vi "main.vi"(8 "error in (no error)":errorcluster, 9 "enable_event":bool, 10 "max_queue_size":i32=10, 11 "references_queue":refnum<queue>) -> (0 "error out":errorcluster)   [LabVIEW 2015, in "repub-dvr_nre.lvlib"]
doc: "This VI is (a) focal point of the module in the event that there is a need to serialize processes or have loops specific to the module that need to run to aid in the modules major functionality."
uses:
  repub-dvr_nre.lvlib
  public/_controls/references.ctl
  private/_controls/input.ctl
  private/_controls/input_command.ctl
  private/_controls/output.ctl
  private/_controls/data.ctl
  public/_controls/configuration.ctl
  lv-recipe-machine/private/_controls/recipe_data.ctl
  lv-recipe-machine/public/_controls/mode.ctl
  lv-recipe-machine/public/_controls/manual_state.ctl
  lv-recipe-machine/public/_controls/automatic_state.ctl
  <userlib>/antonio-alexander/lv-waitgroup/public/_controls/api_waitgroup.ctl
  lv-recipe-machine/public/_controls/transition.ctl
  public/_controls/change.ctl
  public/_controls/status.ctl
  public/_controls/error.ctl
  lv-recipe-machine/lv-recipe-machine.lvlib
  <userlib>/antonio-alexander/lv-waitgroup/lv-waitgroup.lvlib
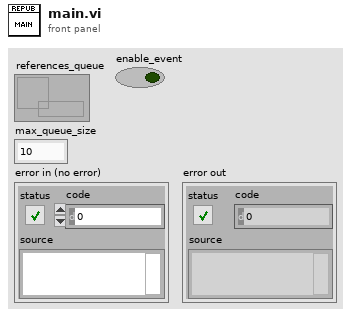
[diagram p1: front panel]
types:
  T1 = typedef "lv-recipe-machine.lvlib/transition.ctl" = cluster{"next_step":string, "data":variant, "error":errorcluster}
  T2 = typedef "repub-dvr_nre.lvlib/references.ctl" = cluster{"semaphore":T3, "input_queue":refnum<queue>, "output_queue":refnum<queue>, "data_dvr":refnum<data-value>, "stop_notifier":refnum<notifier>, "transition_queue":refnum<queue>, "change_in_queue":refnum<queue>, "change_out_queue":refnum<queue>, "status_queue":refnum<queue>, "change_in_event":refnum<user-event>, "change_out_event":refnum<user-event>, "status_event":refnum<user-event>}
  T3 = typedef "Semaphore RefNum" = refnum<k1>
  T4 = typedef "repub-dvr_nre.lvlib/output.ctl" = cluster{"data":variant, "error":errorcluster}
  T5 = typedef "repub-dvr_nre.lvlib/input.ctl" = cluster{"command":T6, "data":variant}
  T6 = typedef "repub-dvr_nre.lvlib/input_command.ctl" = enum8{"<input_command>", "die", "<null>"}
  T7 = typedef "repub-dvr_nre.lvlib/data.ctl" = cluster{"configuration":T8, "working":cluster{"recipe_data":T9, "api_waitgroup":T13}}
  T8 = typedef "repub-dvr_nre.lvlib/configuration.ctl" = cluster{dbl}
  T9 = typedef "lv-recipe-machine.lvlib/recipe_data.ctl" = cluster{"mode":T10, "manual_state":T11, "automatic_state":T12, "step":string, "automatic_recipe":variant, "manual_actions":variant}
  T10 = typedef "lv-recipe-machine.lvlib/mode.ctl" = enum16{"<mode>", "manual", "automatic", "<null>"}
  T11 = typedef "lv-recipe-machine.lvlib/manual_state.ctl" = enum16{"<manual_state>", "failed", "action", "running", "idle", "<null>"}
  T12 = typedef "lv-recipe-machine.lvlib/automatic_state.ctl" = enum16{"<automatic_state>", "failed", "idle", "running", "paused", "transition", "stopped", "<null>"}
  T13 = typedef "lv-waitgroup.lvlib/api_waitgroup.ctl" = cluster{"waitgroups":refnum<data-value>, "waitgroup":string}
  T14 = typedef "repub-dvr_nre.lvlib/status.ctl" = cluster{"mode":T10, "manual_state":T11, "automatic_state":T12, "step":string}
  T15 = typedef "repub-dvr_nre.lvlib/change.ctl" = cluster{"changed":bool, "data":variant}
  T16 = typedef "repub-dvr_nre.lvlib/error.ctl" = enum16{"<error>", "bad_command", "command_queue_timeout", "stop_notifier_timeout", "die_command_timeout", "<null>"}
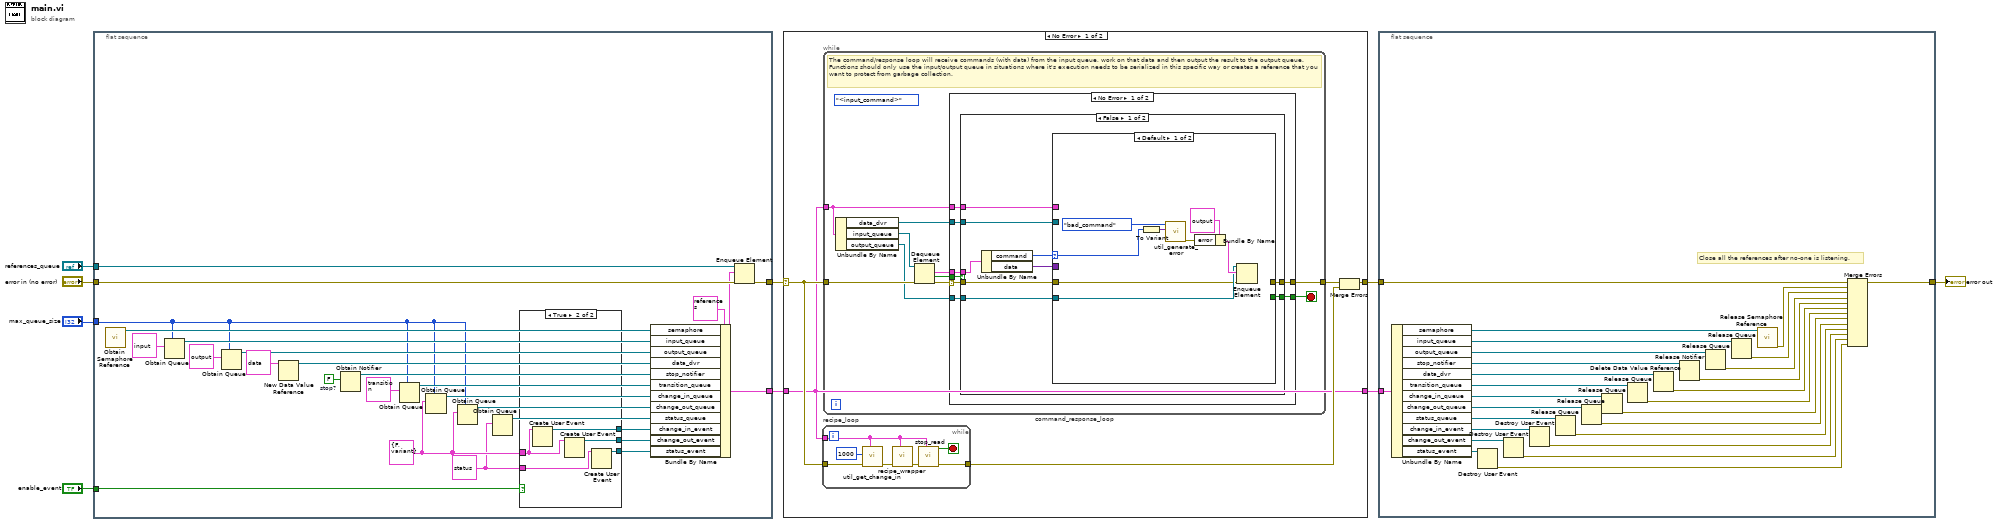
[diagram p0: block diagram]
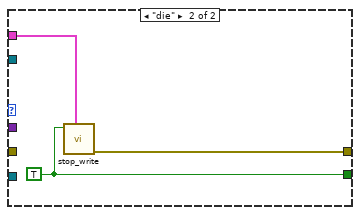
[diagram p3: hidden frame]
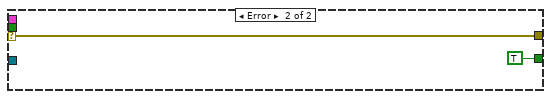
[diagram p5: hidden frame]
diagram:
  n1 = flat-sequence {
    tunnel: "error in (no error)" -> [w25]
    tunnel: "max_queue_size" -> [w13]
    tunnel: "references_queue" -> [w26]
    tunnel: [w24] -> w4
    tunnel: [w23] -> w3
    tunnel: "enable_event" -> [w17]
    frame #0 {
      w10 = T14 {"mode"=enum."<mode>", "manual_state"=enum."<manual_state>", "automatic_state"=enum."<automatic_state>", "step"=""} ("status")
      w18 = T15 {"changed"=FALSE, "data"=variant} ("change")
      w35 = FALSE  # stop?
      n2 = call <vilib>:"Obtain Semaphore Reference.vi"() -> ("semaphore"=w22:T3)  [unwired: 5 in, 2 out]
      n3 = Obtain Queue(max queue size (-1, unlimited)=w13, element data type=T5 {"command"=enum."<input_command>", "data"=variant(cluster{"data":variant} {"data"=variant})} ("input")) -> (queue out=w31:refnum<queue>)  [unwired: 3 in, 2 out]
      n4 = Obtain Queue(max queue size (-1, unlimited)=w13, element data type=T4 {"data"=variant(cluster{"error":errorcluster} {"error"={"status"=FALSE, "code"=0, "source"=""}}), "error"={"status"=FALSE, "code"=0, "source"=""}} ("output")) -> (queue out=w30:refnum<queue>)  [unwired: 3 in, 2 out]
      n5 = New Data Value Reference(data value=T7 {"configuration"={0.0}, "working"={"recipe_data"={"mode"=enum."<mode>", "manual_state"=enum."<manual_state>", "automatic_state"=enum."<automatic_state>", "step"="", "automatic_recipe"=variant, "manual_actions"=variant}, "api_waitgroup"={"waitgroups"=refnum, "waitgroup"=""}}} ("Data")) -> (data value reference=w28:refnum<data-value>)  [unwired: 1 in, 1 out]
      n6 = Obtain Notifier(notification data type=w35) -> (notifier out=w27:refnum<notifier>)  [unwired: 3 in, 2 out]
      n7 = Obtain Queue(max queue size (-1, unlimited)=w13, element data type=T1 {"next_step"="", "data"=variant, "error"={"status"=FALSE, "code"=0, "source"=""}} ("transition")) -> (queue out=w15:refnum<queue>)  [unwired: 3 in, 2 out]
      n8 = Obtain Queue(max queue size (-1, unlimited)=w13, element data type=w18) -> (queue out=w14:refnum<queue>)  [unwired: 3 in, 2 out]
      n9 = Obtain Queue(max queue size (-1, unlimited)=w13, element data type=w18) -> (queue out=w21:refnum<queue>)  [unwired: 3 in, 2 out]
      n10 = Obtain Queue(element data type=w10) -> (queue out=w12:refnum<queue>)  [unwired: 4 in, 2 out]
      n11 = case shown="True" w17 {
        tunnel: [_ w40] -> w20
        tunnel: [_ w39] -> w19
        tunnel: w18 -> [_ w38]
        tunnel: [_ w37] -> w11
        tunnel: w10 -> [_ w36]
        frame False {
        }
        frame True {
          n12 = Create User Event(user event datatype=w38) -> (user event=w40:refnum<user-event>)  [unwired: 1 in, 1 out]
          n13 = Create User Event(user event datatype=w38) -> (user event=w39:refnum<user-event>)  [unwired: 1 in, 1 out]
          n14 = Create User Event(user event datatype=w36) -> (user event=w37:refnum<user-event>)  [unwired: 1 in, 1 out]
        }
      }
      n15 = Bundle By Name(cluster=T2 {"semaphore"=refnum, "input_queue"=refnum, "output_queue"=refnum, "data_dvr"=refnum, "stop_notifier"=refnum, "transition_queue"=refnum, "change_in_queue"=refnum, "change_out_queue"=refnum, "status_queue"=refnum, "change_in_event"=refnum, "change_out_event"=refnum, "status_event"=refnum} ("references"), "semaphore"=w22, "input_queue"=w31, "output_queue"=w30, "data_dvr"=w28, "stop_notifier"=w27, "transition_queue"=w15, "change_in_queue"=w14, "change_out_queue"=w21, "status_queue"=w12, "change_in_event"=w20, "change_out_event"=w19, "status_event"=w11) -> (w23:T2)
      n16 = Enqueue Element(queue=w26, element=w23, error in (no error)=w25) -> (error out=w24:errorcluster)  [unwired: 1 in, 2 out]
    }
  }
  n17 = case shown="No Error" w4 {
    selector: w4 -> [w43 w94]
    tunnel: [w41 w94] -> w7
    tunnel: w3 -> [w42 w93]
    tunnel: [w42 w93] -> w2
    frame No Error {
      n18 = while "recipe_loop" {
        tunnel: w43 -> [w87]
        tunnel: w42 -> [w91]
        tunnel: [w88] -> w45
        stop <- w89 stop-if-true
        n19 = call "util_get_change_in.vi"("references"=w91, "error in (no error)"=w87, "timeout"=1000) -> ("error out"=w86:errorcluster)  [unwired: 6 in, 2 out]
        n20 = call "recipe_wrapper.vi"("references"=w91, "error in (no error)"=w86) -> ("error out"=w90:errorcluster)  [unwired: 9 in]
        n21 = call "stop_read.vi"("references"=w91, "error in (no error)"=w90) -> ("error out"=w88:errorcluster, "stop?"=w89:bool)  [unwired: 8 in]
      }
      n22 = while "command_response_loop" {
        tunnel: w43 -> [w55]
        tunnel: [w51] -> w44
        tunnel: w42 -> [w46]
        stop <- w47 stop-if-true
        (unwired) input_command."<input_command>" ("command")
        # "The command/response loop will receive commands (with data) from the input queue, work on that data and then output the result to the output queue. Functions should only use the input/output queue in situations where it's execution needs to be serialized in this specific way or creates a reference that you want to protect from garbage collection."
        n23 = Unbundle By Name(w46) -> ("data_dvr"=w50:refnum<data-value>, "input_queue"=w49:refnum<queue>, "output_queue"=w48:refnum<queue>)
        n24 = Dequeue Element(queue=w49, error in (no error)=w55) -> (element=w52:T5, timed out?=w54:bool, error out=w53:errorcluster)  [unwired: 1 in, 1 out]
        n25 = case shown="No Error" w53 {
          selector: w53 -> [w62 w84]
          tunnel: w54 -> [w63 _]
          tunnel: w52 -> [w61 _]
          tunnel: [w56 w84] -> w51
          tunnel: w50 -> [w60 _]
          tunnel: w48 -> [w59 _]
          tunnel: [w58 TRUE] -> w47
          tunnel: w46 -> [w57 _]
          frame No Error {
            n26 = case shown="False" w63 {
              tunnel: w62 -> [w66 _]
              tunnel: w61 -> [w72 _]
              tunnel: w60 -> [w70 _]
              tunnel: w59 -> [w69 _]
              tunnel: [w67 _] -> w58
              tunnel: w57 -> [w65 _]
              tunnel: [w64 _] -> w56
              frame False {
                n27 = Unbundle By Name(w72) -> ("command"=w71:T6, "data"=w68:variant)
                n28 = case shown="Default" w71 {
                  selector: w71 -> [w77 _]
                  tunnel: w66 -> [w73 _]
                  tunnel: w70 -> [_ _]
                  tunnel: w69 -> [w74 _]
                  tunnel: w68 -> [_ _]
                  tunnel: [_ w83] -> w67
                  tunnel: w65 -> [_ w81]
                  tunnel: [_ w82] -> w64
                  frame Default {
                    n29 = To Variant(anything=w77) -> (Variant=w76:variant)
                    n30 = call "util_generate_error.vi"("data"=w76, "error"=error."bad_command" ("Error")) -> ("error out"=w79:errorcluster)  [unwired: 9 in]
                    n31 = Bundle By Name(cluster=T4 {"data"=variant(cluster{"error":errorcluster} {"error"={"status"=FALSE, "code"=0, "source"=""}}), "error"={"status"=FALSE, "code"=0, "source"=""}} ("element"), "error"=w79) -> (w80:T4)
                    n32 = Enqueue Element(queue=w74, element=w80, error in (no error)=w73) -> ()  [unwired: 1 in, 3 out]
                  }
                  frame "die" {
                    w83 = TRUE
                    n33 = call "stop_write.vi"("references"=w81, "stop"=w83) -> ("error out"=w82:errorcluster)  [unwired: 9 in]
                  }
                }
              }
              frame True {
              }
            }
          }
          frame Error {
          }
        }
      }
      n34 = Merge Errors(w44, w45) -> (w41:errorcluster)
    }
    frame Error {
    }
  }
  n35 = flat-sequence {
    tunnel: [w116] -> w8
    tunnel: w7 -> [w121]
    tunnel: w2 -> [w114]
    frame #0 {
      # "Close all the references after no-one is listening."
      n36 = Unbundle By Name(w114) -> ("semaphore"=w110:T3, "input_queue"=w119:refnum<queue>, "output_queue"=w120:refnum<queue>, "stop_notifier"=w118:refnum<notifier>, "data_dvr"=w117:refnum<data-value>, "transition_queue"=w100:refnum<queue>, "change_in_queue"=w106:refnum<queue>, "change_out_queue"=w105:refnum<queue>, "status_queue"=w97:refnum<queue>, "change_in_event"=w108:refnum<user-event>, "change_out_event"=w107:refnum<user-event>, "status_event"=w98:refnum<user-event>)
      n37 = Destroy User Event(user event=w98) -> (error out=w95:errorcluster)  [unwired: 1 in]
      n38 = Destroy User Event(user event=w107) -> (error out=w101:errorcluster)  [unwired: 1 in]
      n39 = Destroy User Event(user event=w108) -> (error out=w102:errorcluster)  [unwired: 1 in]
      n40 = Release Queue(queue=w97) -> (error out=w96:errorcluster)  [unwired: 2 in, 2 out]
      n41 = Release Queue(queue=w105) -> (error out=w103:errorcluster)  [unwired: 2 in, 2 out]
      n42 = Release Queue(queue=w106) -> (error out=w104:errorcluster)  [unwired: 2 in, 2 out]
      n43 = Release Queue(queue=w100) -> (error out=w99:errorcluster)  [unwired: 2 in, 2 out]
      n44 = Delete Data Value Reference(data value reference=w117) -> (error out=w112:errorcluster)  [unwired: 1 in, 1 out]
      n45 = Release Notifier(notifier=w118) -> (error out=w113:errorcluster)  [unwired: 2 in, 2 out]
      n46 = Release Queue(queue=w120) -> (error out=w115:errorcluster)  [unwired: 2 in, 2 out]
      n47 = Release Queue(queue=w119) -> (error out=w111:errorcluster)  [unwired: 2 in, 2 out]
      n48 = call <vilib>:"Release Semaphore Reference.vi"("semaphore"=w110) -> ("error out"=w109:errorcluster)  [unwired: 9 in, 1 out]
      n49 = Merge Errors(w121, w109, w111, w115, w113, w112, w99, w104, w103, w96, w102, w101, w95) -> (w116:errorcluster)
    }
  }
  "error out" <- w8
